vi "Error Top Level.vi"(8 "error in (no error)":errorcluster) -> (0 "error out":errorcluster)   [LabVIEW 2020, in "Error Handler.lvlib"]
uses:
  Error Handler.lvlib
  Private Controls/Module Action.ctl
  Private Controls/Error React.ctl
  Public Controls/Module Data Cluster.ctl
  252a235d-993b-4b77-be99-5936f81e7a50.vi
  b2557411-5cff-4c84-9b89-16ab07a25453.vi
  27c827a8-6ce2-46ff-b742-8397f53ceddc.vi
  e3555320-3669-4681-98ae-afe808cba037.vi
  16cb41ff-8f3c-4f22-bc48-50ffacbfc1d7.vi
  <vilib>/Utility/error.llb/Clear Errors.vi
  Architecture Support/Architecture Support.lvlib
  UI/UI.lvlib
panel:
  out "Error Response":T1
  out "Action":T2
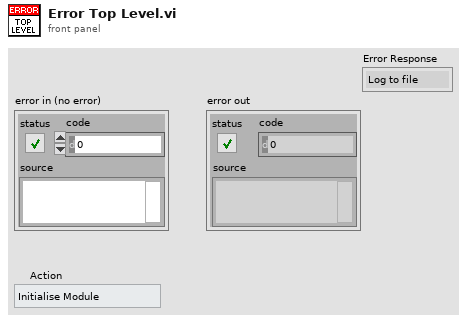
[diagram p1: front panel]
types:
  T1 = typedef "Error Handler.lvlib/Error React.ctl" = enum16{"Log to file", "Prompt User", "Prompt & Log", "Abort Code", "Ignore"}
  T2 = typedef "Error Handler.lvlib/Module Action.ctl" = enum16{"Initialise Module", "Modify Reaction to Error", "Log to File", "Prompt User", "External Error", "Internal Error", "Exit"}
  T3 = typedef "Error Handler.lvlib/Module Data Cluster.ctl" = cluster{"Error Response":T1, "Error Log Refnum Out":refnum<file>}
  T4 = enum16{"open", "replace", "create", "open or create", "replace or create", "replace or create with confirmation"}
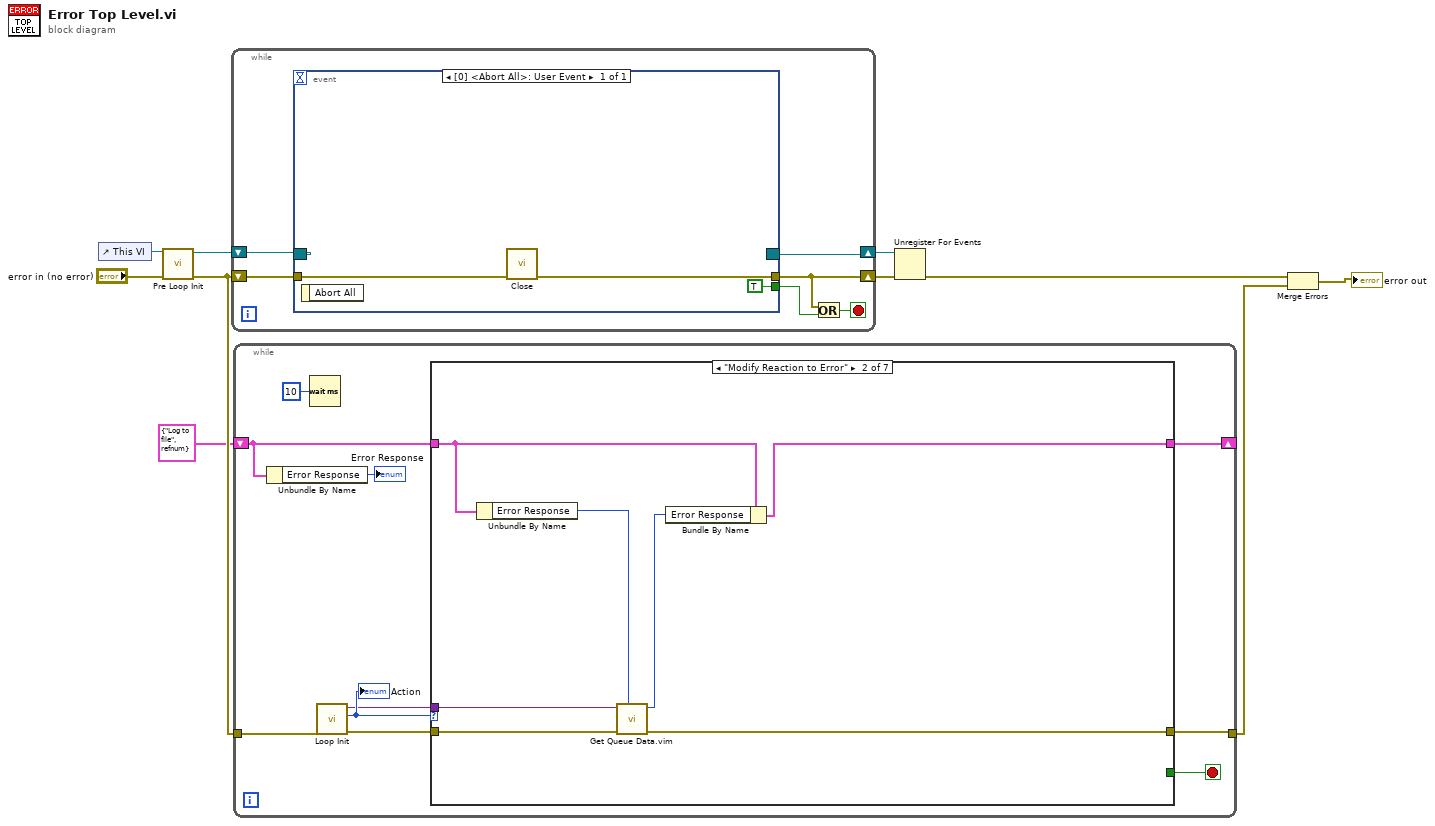
[diagram p0: block diagram]
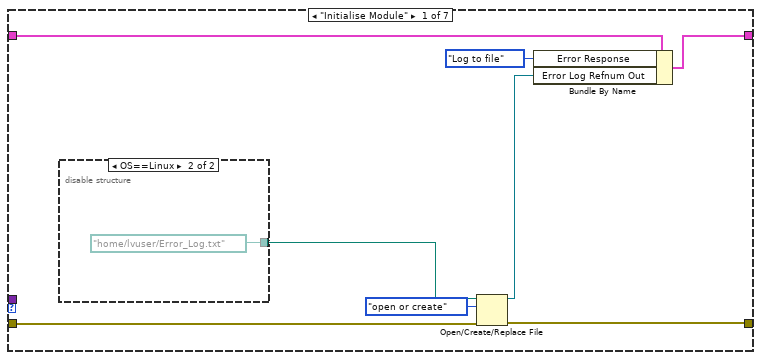
[diagram p2: hidden frame]
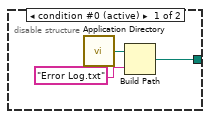
[diagram p3: hidden frame]
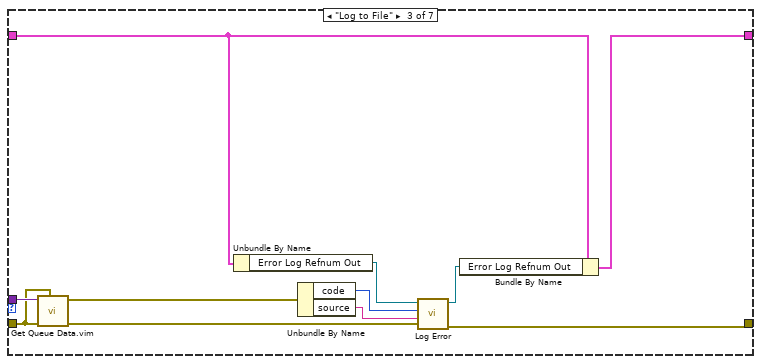
[diagram p4: hidden frame]
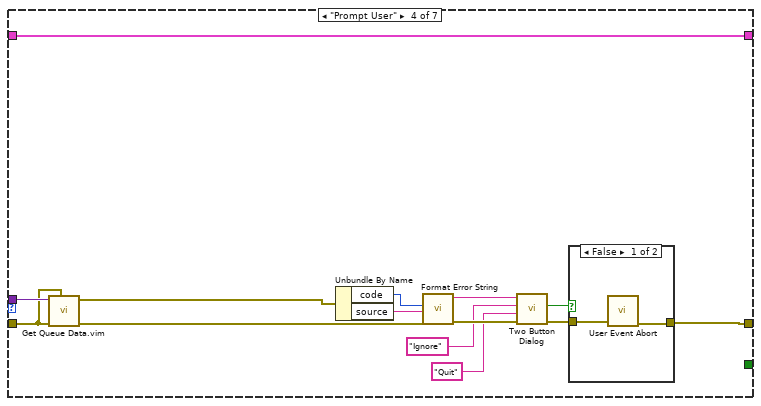
[diagram p5: hidden frame]
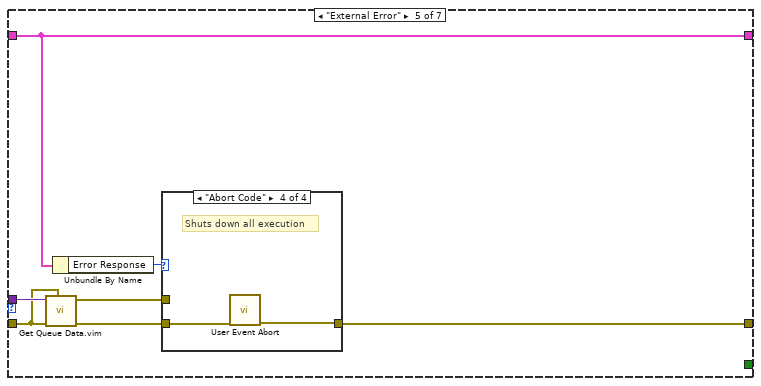
[diagram p7: hidden frame]
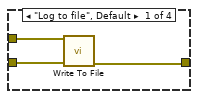
[diagram p8: hidden frame]
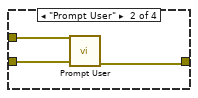
[diagram p9: hidden frame]
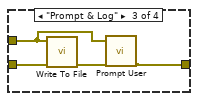
[diagram p10: hidden frame]
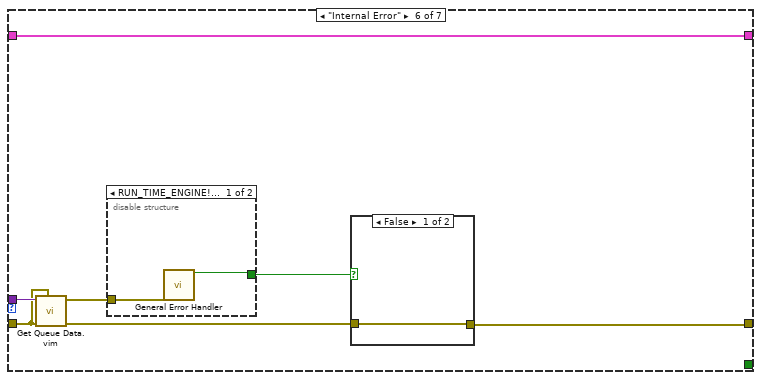
[diagram p11: hidden frame]
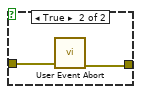
[diagram p12: hidden frame]
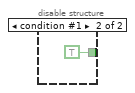
[diagram p13: hidden frame]
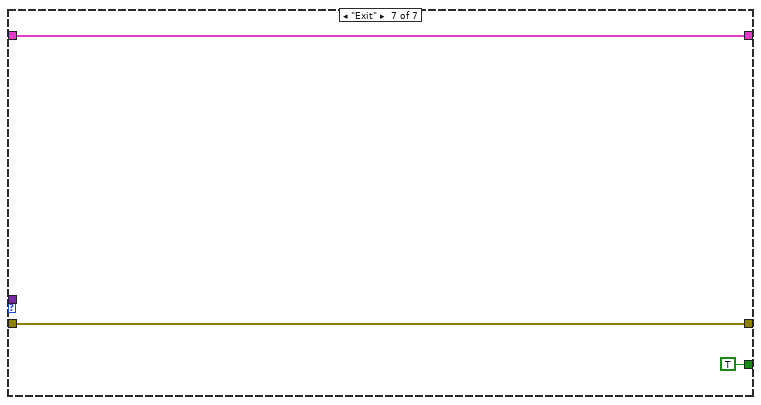
[diagram p14: hidden frame]
diagram:
  n1 = control-ref of="This VI"() -> (w4:refnum<vi>)
  n2 = call "Pre Loop Init.vi"("error in (no error)"="error in (no error)", "Ref In"=w4) -> ("error out"=w6:errorcluster, "Event Registration Refnum"=w1:refnum<event-registration>)  [unwired: 8 in]
  n3 = while {
    shift-right: [w13] -> w9
    shift-left: w6 -> [w12]
    shift-right: [w15] -> w5
    shift-left: w1 -> [w16]
    stop <- w14 stop-if-true
    n4 = event shown="[0] <Abort All>: User Event" {
      selector: w16 -> [_]
      dyn-events: [_] -> w15
      timeout: _ -> [_]
      tunnel: [w18] -> w13
      tunnel: w12 -> [w19]
      tunnel: [TRUE] -> w11
      event User Event {
        n5 = event-data() -> ()  [unwired: 1 in, 1 out]
        n6 = call "Close.vi"("error in (no error)"=w19) -> ("error out"=w18:errorcluster)  [unwired: 10 in]
      }
    }
    n7 = Or(x=w13, y=w11) -> (x .or. y?=w14:bool)
  }
  n8 = while {
    shift-right: [w24] -> _
    shift-left: T3 {"Error Response"=enum."Log to file", "Error Log Refnum Out"=refnum} ("Module Data Cluster") -> [w21]
    tunnel: w6 -> [w28]
    tunnel: [w25] -> w7
    stop <- w23 stop-if-true
    n9 = Unbundle By Name(w21) -> ("Error Response"=→"Error Response":T1)
    n10 = Wait (ms)(milliseconds to wait=u32 10) -> ()  [unwired: 1 out]
    n11 = call "Loop Init.vi"("error in (no error)"=w28) -> ("error out"=w26:errorcluster, "Action"=w27:T2, "Data"=w22:variant)  [unwired: 8 in]
    "Action" <- w27
    n12 = case shown="\"Modify Reaction to Error\"" w27 {
      tunnel: w26 -> [w35 w48 w55 w72 w77 w100 w109]
      tunnel: [w30 w46 w57 w67 w81 w98 w109] -> w25
      tunnel: w21 -> [w37 w43 w49 w60 w80 w102 w111]
      tunnel: [w36 w42 w50 w60 w80 w102 w111] -> w24
      tunnel: [_ _ _ _ _ _ TRUE] -> w23
      tunnel: w22 -> [_ w47 w59 w73 w83 w101 _]
      frame "Initialise Module" {
        n13 = disable-structure shown="OS==Linux" {
          disable-tunnel: [w38 path "/home/lvuser/Error_Log.txt" ("appended path")] -> w34
          frame condition #0 (active) {
            n14 = call <vilib>:"Application Directory.vi"() -> ("Application Directory"=w40:path)
            n15 = Build Path(base path=w40, name or relative path="Error Log.txt") -> (appended path=w38:path)
          }
          frame condition #1 {
          }
        }
        n16 = Open/Create/Replace File(file path (use dialog)=w34, error in=w35, operation (0:open)=T4."open or create") -> (refnum out=w33:refnum<file>, error out=w30:errorcluster)  [unwired: 3 in, 1 out]
        n17 = Bundle By Name(cluster=w37, "Error Response"=Error_React."Log to file", "Error Log Refnum Out"=w33) -> (w36:T3)
      }
      frame "Modify Reaction to Error" {
        n18 = Unbundle By Name(w43) -> ("Error Response"=w45:T1)
        n19 = call "Get Queue Data.vim"("Default Value"=w45, "error in"=w48, "Variant"=w47) -> ("error out"=w46:errorcluster, "Module Data"=w44:T1)  [unwired: 7 in]
        n20 = Bundle By Name(cluster=w43, "Error Response"=w44) -> (w42:T3)
      }
      frame "Log to File" {
        n21 = call "Get Queue Data.vim"("Default Value"=w55, "error in"=w55, "Variant"=w59) -> ("error out"=w58:errorcluster, "Module Data"=w56:errorcluster)  [unwired: 7 in]
        n22 = Unbundle By Name(w49) -> ("Error Log Refnum Out"=w52:refnum<file>)
        n23 = Unbundle By Name(w56) -> ("code"=w53:i32, "source"=w54:string)
        n24 = call "Log Error.vi"("error in (no error)"=w58, "Source"=w54, "Code"=w53, "Error Log Refnum In"=w52) -> ("error out"=w57:errorcluster, "Error Log Refnum Out"=w51:refnum<file>)  [unwired: 6 in]
        n25 = Bundle By Name(cluster=w49, "Error Log Refnum Out"=w51) -> (w50:T3)
      }
      frame "Prompt User" {
        n26 = call "Get Queue Data.vim"("Default Value"=w72, "error in"=w72, "Variant"=w73) -> ("error out"=w70:errorcluster, "Module Data"=w71:errorcluster)  [unwired: 7 in]
        n27 = Unbundle By Name(w71) -> ("code"=w68:i32, "source"=w69:string)
        n28 = call "Format Error String.vi"("error in (no error)"=w70, "Source"=w69, "Code"=w68) -> ("error out"=w66:errorcluster, "Error String"=w64:string)  [unwired: 7 in]
        n29 = call "Two Button Dialog.vi"("error in (no error)"=w66, "Retry Text In"="Quit", "Cancel Text In"="Ignore", "Message Text In"=w64) -> ("error out"=w65:errorcluster, "Continue?"=w61:bool)  [unwired: 6 in]
        n30 = case shown="False" w61 {
          tunnel: w65 -> [w75 w76]
          tunnel: [w74 w76] -> w67
          frame False {
            n31 = call "User Event Abort.vi"("error in (no error)"=w75) -> ("error out"=w74:errorcluster)  [unwired: 9 in, 1 out]
          }
          frame True {
          }
        }
      }
      frame "External Error" {
        n32 = call "Get Queue Data.vim"("Default Value"=w77, "error in"=w77, "Variant"=w83) -> ("error out"=w82:errorcluster, "Module Data"=w78:errorcluster)  [unwired: 7 in]
        n33 = Unbundle By Name(w80) -> ("Error Response"=w79:T1)
        n34 = case shown="\"Abort Code\"" w79 {
          tunnel: w82 -> [w86 w88 w93 w95]
          tunnel: [w85 w87 w91 w94] -> w81
          tunnel: w78 -> [w84 w89 w90 _]
          frame "Log to file", Default {
            n35 = call "Write To File.vi"("error in (no error)"=w86, "Data"=w84) -> ("error out"=w85:errorcluster)  [unwired: 9 in]
          }
          frame "Prompt User" {
            n36 = call "Prompt User.vi"("error in (no error)"=w88, "Data"=w89) -> ("error out"=w87:errorcluster)  [unwired: 9 in]
          }
          frame "Prompt & Log" {
            n37 = call "Write To File.vi"("error in (no error)"=w93, "Data"=w90) -> ("error out"=w92:errorcluster)  [unwired: 9 in]
            n38 = call "Prompt User.vi"("error in (no error)"=w92, "Data"=w90) -> ("error out"=w91:errorcluster)  [unwired: 9 in]
          }
          frame "Abort Code" {
            # "Shuts down all execution"
            n39 = call "User Event Abort.vi"("error in (no error)"=w95) -> ("error out"=w94:errorcluster)  [unwired: 9 in, 1 out]
          }
        }
      }
      frame "Internal Error" {
        n40 = call "Get Queue Data.vim"("Default Value"=w100, "error in"=w100, "Variant"=w101) -> ("error out"=w99:errorcluster, "Module Data"=w96:errorcluster)  [unwired: 7 in]
        n41 = disable-structure shown="RUN_TIME_ENGINE!=True" {
          disable-tunnel: [w106 TRUE] -> w97
          disable-tunnel: w96 -> [w107 _]
          frame condition #0 (active) {
            n42 = call <vilib>:"General Error Handler.vi"("error in (no error)"=w107) -> ("error?"=w106:bool)  [unwired: 10 in, 4 out]
          }
          frame condition #1 {
          }
        }
        n43 = case shown="False" w97 {
          tunnel: w99 -> [w103 w105]
          tunnel: [w103 w104] -> w98
          frame False {
          }
          frame True {
            n44 = call "User Event Abort.vi"("error in (no error)"=w105) -> ("error out"=w104:errorcluster)  [unwired: 9 in, 1 out]
          }
        }
      }
      frame "Exit" {
      }
    }
  }
  n45 = Unregister For Events(event registration refnum=w5, error in=w9) -> (error out=w8:errorcluster)
  n46 = Merge Errors(w8, w7) -> (→"error out":errorcluster)
